vi "AvantesGetSpectrumFGV.vi"(8 "error in":errorcluster, 10 "Set_Get":enum16{"Set", "Get"}(ring), 11 "in":dbl[][](graph)) -> (0 "error out":errorcluster, 3 "out":dbl[][](graph))   [LabVIEW 2010]
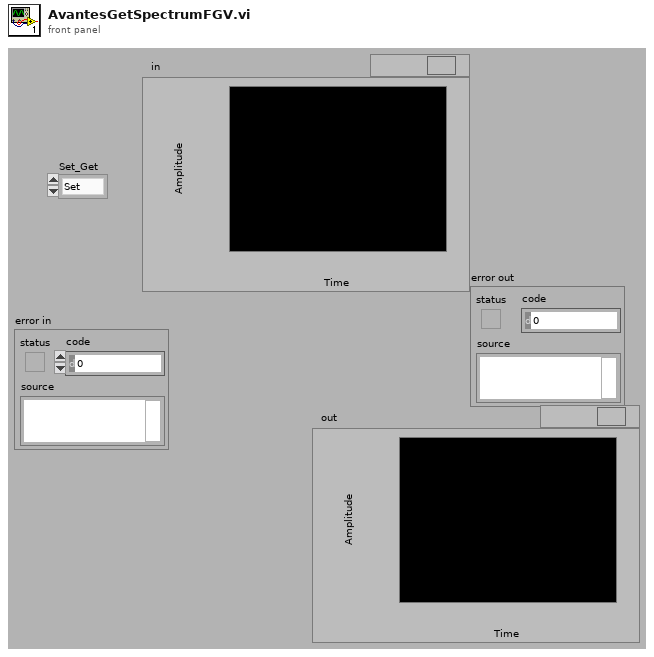
[diagram p1: front panel]
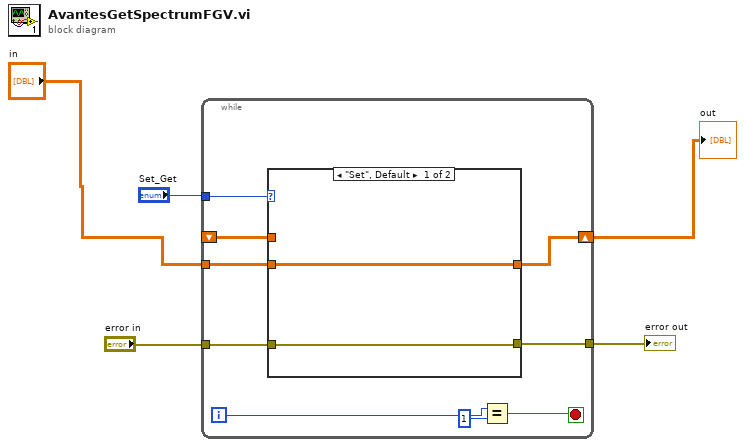
[diagram p0: block diagram]
diagram:
  n1 = while {
    tunnel: "Set_Get" -> [w14]
    tunnel: "in" -> [w13]
    shift-right: [w12] -> w2
    shift-left: _ -> [w11]
    tunnel: [w7] -> w4
    tunnel: "error in" -> [w6]
    i -> [w9]
    stop <- w10 stop-if-true
    n2 = case shown="\"Set\", Default" w14 {
      tunnel: w13 -> [w16 _]
      tunnel: [w16 w17] -> w12
      tunnel: w11 -> [_ w17]
      tunnel: [w15 _] -> w7
      tunnel: w6 -> [w15 _]
      frame "Set", Default {
      }
      frame "Get" {
      }
    }
    n3 = Equal?(x=w9, y=1) -> (x = y?=w10:bool)
  }
  "error out" <- w4
  "out" <- w2
